vi "Fetch Single Measurement (Voltage Harmonics).vi"(0 "VISA resource name":refnum<visa-resource-name>, 7 "Harmonic Order (1)":u8=1, 9 "Phase Order (1)":u8=1, 11 "error in (no error)":errorcluster) -> (3 "Total Voltage Harmonic Distortion":dbl, 4 "VISA resource name out":refnum<visa-resource-name>, 8 "Nth Voltage Harmonic Amplitude":dbl, 10 "Nth Voltage Harmonic Phase":dbl, 15 "error out":errorcluster)   [LabVIEW 2020, in "Agilent 681x Series.lvlib"]
doc: "Fetches and returns the selected order harmonic amplitude and phase measurements, and the total harmonic distortion.\n\n<B>Note:</B>\n\nUse this VI only with other low-level VIs. The high-level VIs automatically incorporate this functionality. This VI does not check the instrument status. If you want to check the instrument status, call the Error Query VI at the conclusion of the sequence."
uses:
  <instrlib>/Agilent 681x Series/Agilent 681x Series.lvlib
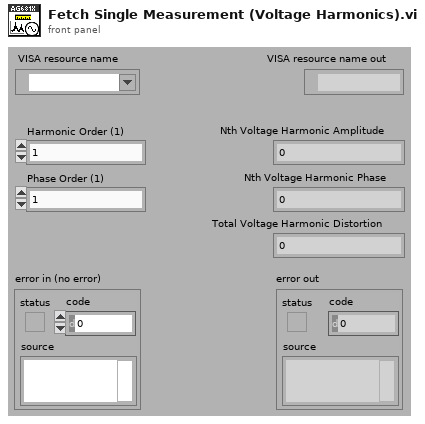
[diagram p1: front panel]
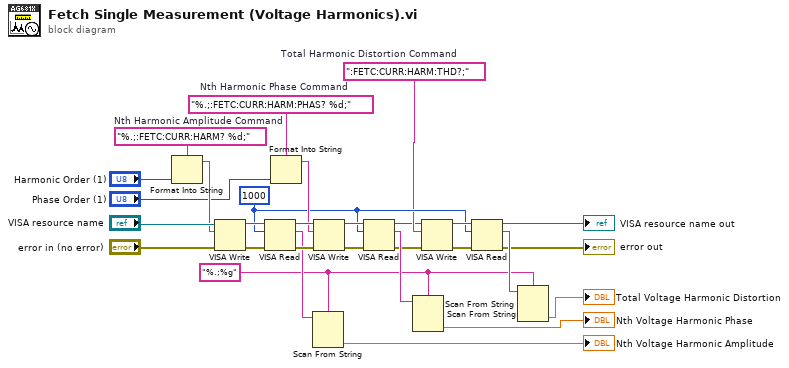
[diagram p0: block diagram]
diagram:
  w6 = "%.;%g" ("format string")
  w18 = "%.;:FETC:CURR:HARM:PHAS? %d;"  # Nth Harmonic Phase Command
  w19 = "%.;:FETC:CURR:HARM? %d;"  # Nth Harmonic Amplitude Command
  w13 = u32 1000 ("byte count")
  w12 = ":FETC:CURR:HARM:THD?;"  # Total Harmonic Distortion Command
  n1 = Format Into String(format string=w19, "Harmonic Order (1)") -> (resulting string=w16:string)  [unwired: 2 in, 1 out]
  n2 = VISA Write(VISA resource name="VISA resource name", write buffer=w16, error in (no error)="error in (no error)") -> (VISA resource name out=w26:refnum<visa-resource-name>, error out=w27:errorcluster)  [unwired: 1 out]
  n3 = VISA Read(VISA resource name=w26, byte count=w13, error in (no error)=w27) -> (VISA resource name out=w22:refnum<visa-resource-name>, read buffer=w7:string, error out=w23:errorcluster)  [unwired: 1 out]
  n4 = Format Into String(format string=w18, "Phase Order (1)") -> (resulting string=w15:string)  [unwired: 2 in, 1 out]
  n5 = Scan From String(format string=w6, input string=w7) -> (output 1=→"Nth Voltage Harmonic Amplitude":dbl)  [unwired: 3 in, 3 out]
  n6 = VISA Write(VISA resource name=w22, write buffer=w15, error in (no error)=w23) -> (VISA resource name out=w25:refnum<visa-resource-name>, error out=w24:errorcluster)  [unwired: 1 out]
  n7 = VISA Read(VISA resource name=w25, byte count=w13, error in (no error)=w24) -> (VISA resource name out=w1:refnum<visa-resource-name>, read buffer=w9:string, error out=w2:errorcluster)  [unwired: 1 out]
  n8 = Scan From String(format string=w6, input string=w9) -> (output 1=→"Nth Voltage Harmonic Phase":dbl)  [unwired: 3 in, 3 out]
  n9 = VISA Write(VISA resource name=w1, write buffer=w12, error in (no error)=w2) -> (VISA resource name out=w21:refnum<visa-resource-name>, error out=w20:errorcluster)  [unwired: 1 out]
  n10 = VISA Read(VISA resource name=w21, byte count=w13, error in (no error)=w20) -> (VISA resource name out=→"VISA resource name out":refnum<visa-resource-name>, read buffer=w11:string, error out=→"error out":errorcluster)  [unwired: 1 out]
  n11 = Scan From String(format string=w6, input string=w11) -> (output 1=→"Total Voltage Harmonic Distortion":dbl)  [unwired: 3 in, 3 out]
